vi "Test Launcher.vi"   [LabVIEW 2016, in "Optimization Framework Test.lvlib"]
uses:
  Optimization Framework Test.lvlib
  Optimization Test/Optimization Test.lvclass
  C:/Program Files (x86)/National Instruments/LabVIEW 2016/vi.lib/ActorFramework/Actor/Actor.lvclass
  <vilib>/ActorFramework/Actor/Actor.lvclass
panel:
  # "Launches test of Optimization Framework"
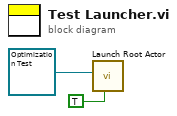
[diagram p0: block diagram]
diagram:
  n1 = call <vilib>:"Launch Root Actor.vi"("Open Actor Core front panel? (F)"=TRUE, "Actor"=refnum<class "Optimization Test.lvclass"> refnum ("Optimization Framework Test.lvlib:Optimization Test.lvclass")) -> ()  [unwired: 8 in, 2 out]
